vi "LarsLab4.vi"() -> ()   [LabVIEW 2010]
panel:
  in  "Ring":u16(ring)
  in  "BoardNumber":dbl
  in  "Channel":dbl
  in  "stop":bool
  out "Waveform Chart":u16(graph)
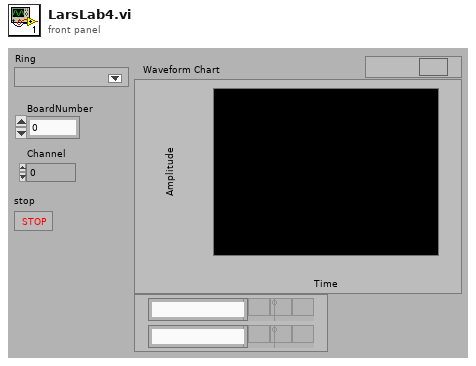
[diagram p1: front panel]
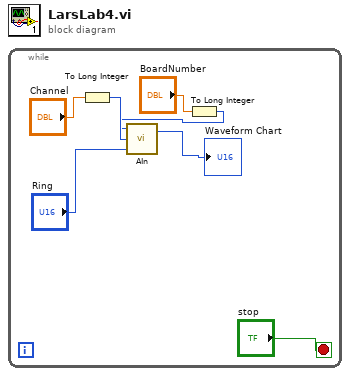
[diagram p0: block diagram]
diagram:
  n1 = while {
    stop <- "stop" stop-if-true
    n2 = To Long Integer(number="Channel") -> (32bit integer=w4:i32)
    n3 = To Long Integer(number="BoardNumber") -> (32bit integer=w2:i32)
    n4 = call <menus>:"AIn.VI"("Range"="Ring", "Channel"=w4, "BoardNum"=w2) -> ("DataValue"=→"Waveform Chart":u16)  [unwired: 1 out]
  }
